vi "Is name unique.vi"(8 "error in (no error)":errorcluster, 10 "Name":string, 11 "Node Ptr":u64 format="%.0x") -> (0 "error out":errorcluster, 1 "Is name unique?":bool, 3 "Node Ptr out":u64 format="%.0x")   [LabVIEW 2013, in "SLSC configuration System Explorer.lvlib"]
uses:
  SLSC configuration System Explorer.lvlib
  <vilib>/NI Veristand/Custom Device API/Custom Device API.lvlib
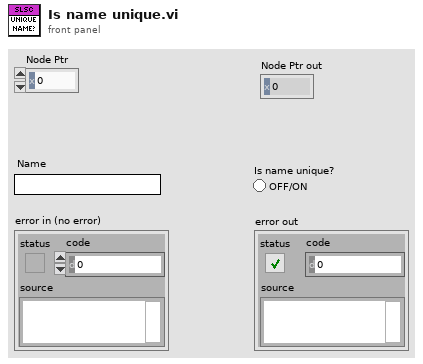
[diagram p1: front panel]
types:
  T1 = typedef "Custom Device API.lvlib/Custom Device Item Ref.ctl" = u64
  T2 = typedef "Custom Device API.lvlib/Custom Device Item Info.ctl" = cluster{"Name":string, "Is Channel":bool, "GUID":string, "Is Waveform":bool}
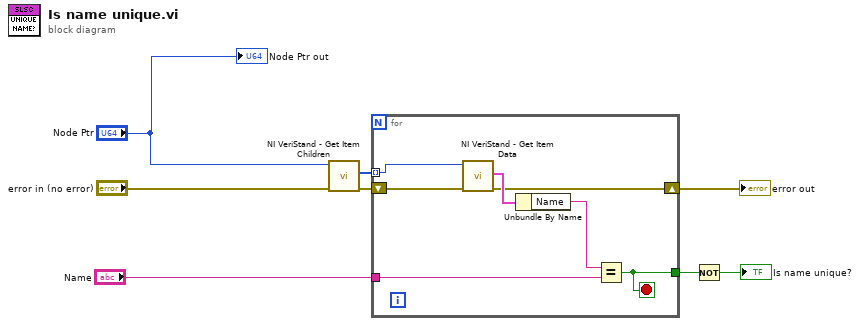
[diagram p0: block diagram]
diagram:
  n1 = call <vilib>:"NI VeriStand - Get Item Children.vi"("error in (no error)"="error in (no error)", "Item Ref in"="Node Ptr") -> ("error out"=w4:errorcluster, "Child Refs"=w2:T1[])  [unwired: 6 in, 2 out]
  n2 = for {
    shift-right: [w12] -> w1
    shift-left: w4 -> [w9]
    tunnel: "Name" -> [w14]
    tunnel: [w11] -> w6
    tunnel: w2 -> [w10] mode=indexing
    stop <- w11 stop-if-true
    n3 = call <vilib>:"NI VeriStand - Get Item Data.vi"("error in (no error)"=w9, "Item Ref in"=w10) -> ("error out"=w12:errorcluster, "Item Info"=w15:T2)  [unwired: 8 out]
    n4 = Unbundle By Name(w15) -> ("Name"=w13:string)
    n5 = Equal?(x=w13, y=w14) -> (x = y?=w11:bool)
  }
  "error out" <- w1
  n6 = Not(x=w6) -> (.not. x?=→"Is name unique?":bool)
  "Node Ptr out" <- "Node Ptr"
